vi "Send-heartbeat.vi"(8 "error in (no error)":errorcluster, 11 "Client in":T1) -> (0 "error out":errorcluster, 3 "Client out":T1)   [LabVIEW 2013, in "CameraVision.lvlib" / "CV-Client.lvclass"]
doc: "Wrapper function for sending the specific 'Hearbeat' type message.\nThis function creates and immediately sends a heartbeat message to the server, using the configuration of the client object."
uses:
  CV-Client.lvclass
  Object-reference.ctl
  CV-Client.lvclass/CV-Client.ctl
  SA-SLMAPI/Sources/Heartbeat/Heartbeat.lvclass
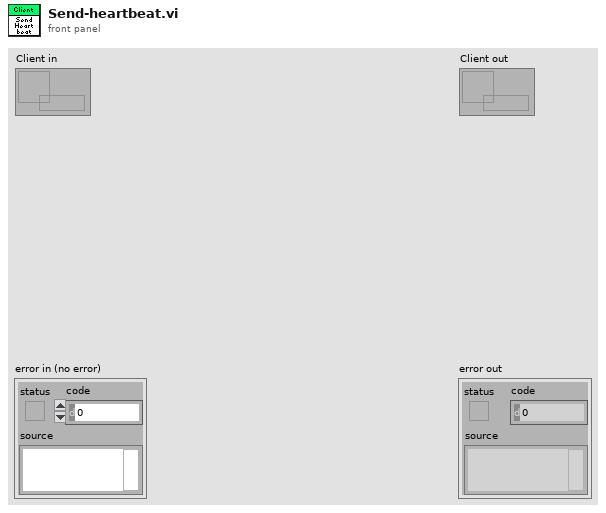
[diagram p1: front panel]
types:
  T1 = typedef "CameraVision.lvlib/CV-Client.lvclass/Object-reference.ctl" = refnum<data-value>
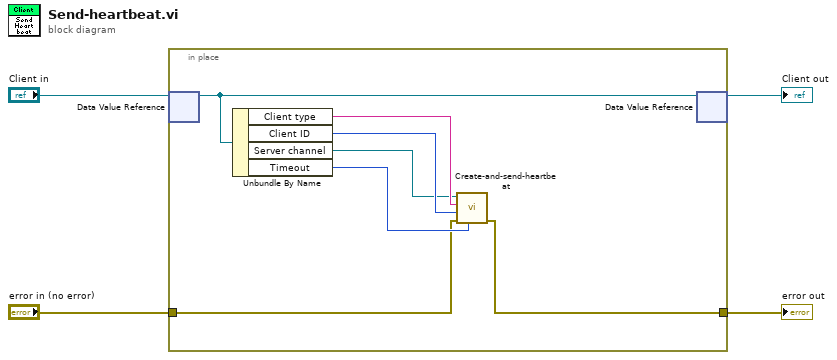
[diagram p0: block diagram]
diagram:
  n1 = in-place {
    in-place-border: "error in (no error)" -> [w7]
    in-place-border: [w5] -> w3
    n2 = in-place-dvr #1("Client in") -> (w6:refnum<class "CV-Client.lvclass">)  [unwired: 1 out]
    n3 = Unbundle By Name(w6) -> ("Client type"=w11:string, "Client ID"=w10:i32, "Server channel"=w9:refnum<queue>, "Timeout"=w8:i32)
    n4 = call "Create-and-send-heartbeat.vi"("Timeout"=w8, "error in (no error)"=w7, "Sender ID"=w10, "Sender"=w11, "Server channel"=w9) -> ("error out"=w5:errorcluster)  [unwired: 6 in]
    n5 = in-place-dvr #1(w6) -> (→"Client out":T1)  [unwired: 1 out]
  }
  "error out" <- w3
